vi "Unpack 32 i12s held in 24 i16s_lvfpga debug.vi"(8 "error in":errorcluster, 9 "destination i16 array":i16[](array[numeric])=[0, 16, 32, 48, 64, 80, 96, 112, 0, 0, 0, 0, 0, 0, 0, 0, 2064, 2320, 2576, 2832, 3088, 3344, 3600, 3856, 256, 256, 256, 256, 256, 256, 256, 256] format="%016b", 10 "packed i12s":i16[](array[numeric])=[0, 16, 32, 48, 64, 80, 96, 112, 2049, 2305, 2561, 2817, 3073, 3329, 3585, 3841, 24, 4121, 8218, 12315, 16412, 20509, 24606, 28703] format="%016b") -> (0 "error out":errorcluster, 1 "destination i16 array out":i16[](array[numeric])=[0, 16, 32, 48, 64, 80, 96, 112, 128, 144, 160, 176, 192, 208, 224, 240, -32768, -28656, -24544, -20432, -16320, -12208, -8096, -3984, 0, 256, 512, 768, 1024, 1280, 1536, 1792] format="%016b")   [LabVIEW 2012]
panel:
  out "destination i16 array (decimal)":i16[](array[numeric])
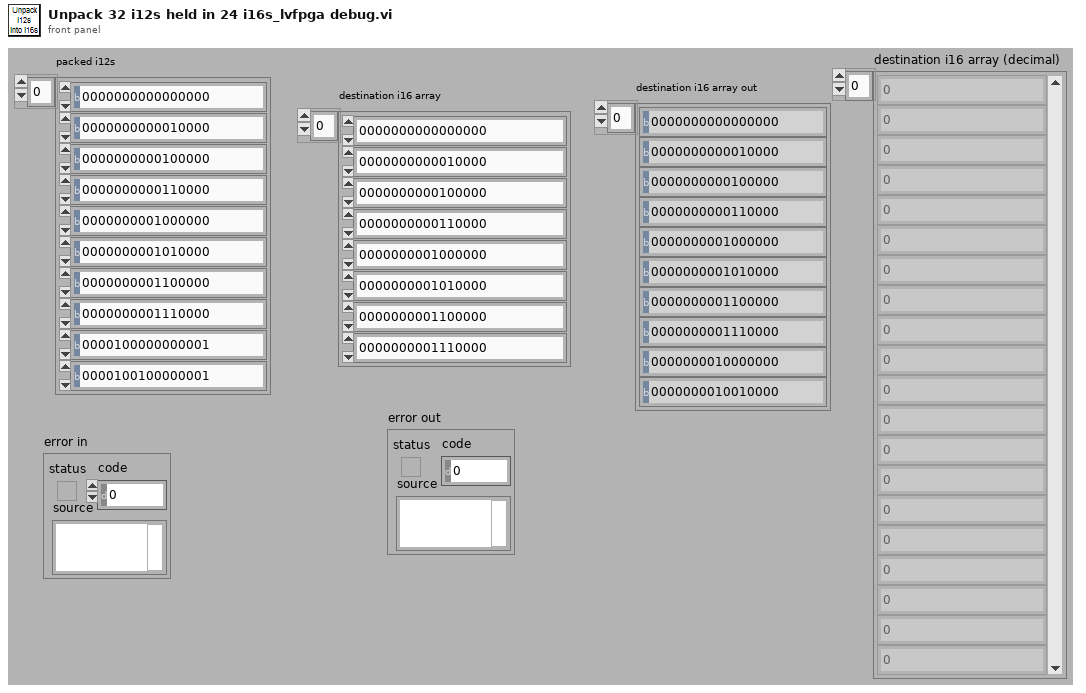
[diagram p1: front panel]
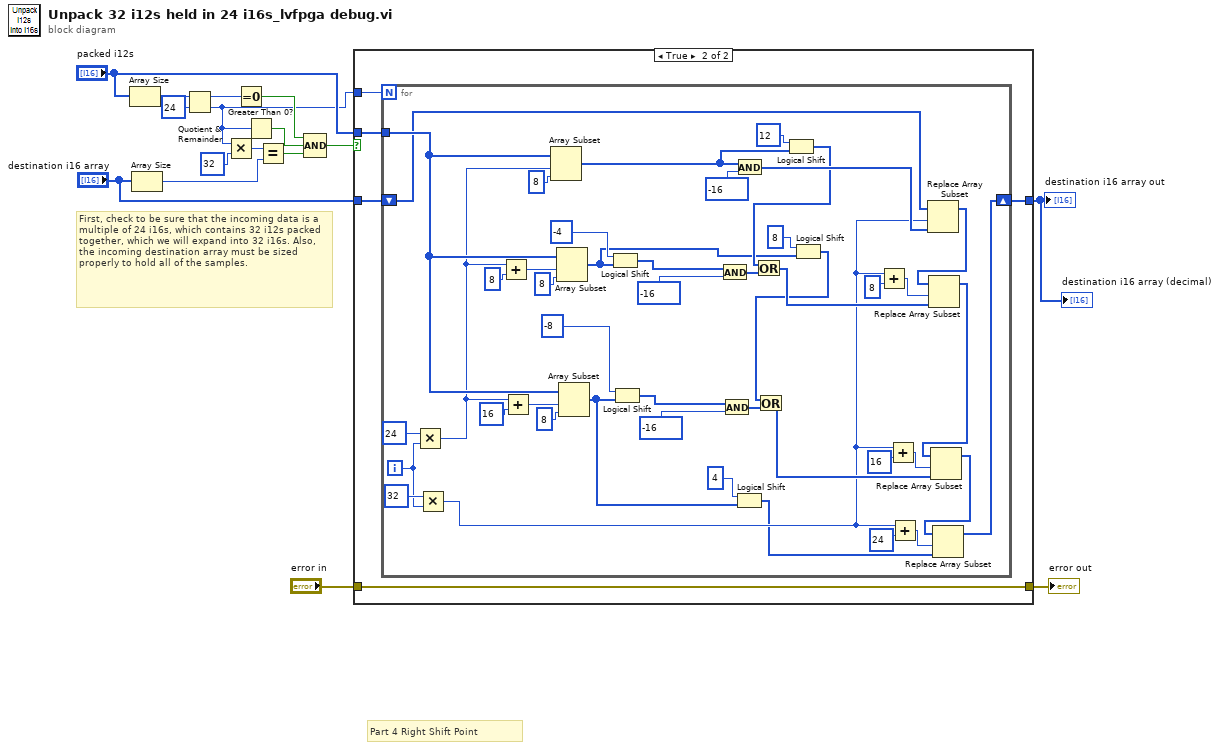
[diagram p0: block diagram]
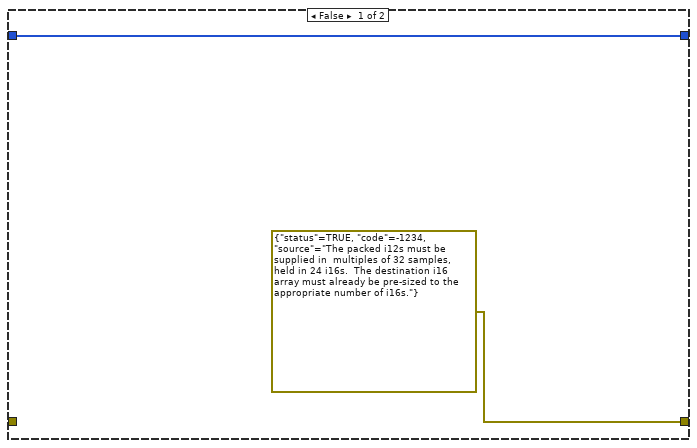
[diagram p2: hidden frame]
diagram:
  # "Part 4 Right Shift Point"
  # "First, check to be sure that the incoming data is a multiple of 24 i16s, which contains 32 i12s packed together, which we will expand into 32 i16s. Also, the incoming destination array must be sized properly to hold all of the samples."
  n1 = Array Size(array="packed i12s") -> (size(s)=w6:i32)
  n2 = Array Size(array="destination i16 array") -> (size(s)=w12:i32)
  n3 = Quotient & Remainder(x=w6, y=24) -> (x-y*floor(x/y)=w16:i32, floor(x/y)=w5:i32)
  n4 = Multiply(x=w5, y=32) -> (x*y=w13:i32)
  n5 = Equal To 0?(x=w16) -> (x = 0?=w11:bool)
  n6 = Greater Than 0?(x=w5) -> (x > 0?=w10:bool)
  n7 = Equal?(x=w13, y=w12) -> (x = y?=w9:bool)
  n8 = Compound Arithmetic op=AND(w11, w10, w9) -> (w7:bool)
  n9 = case shown="True" w7 {
    tunnel: "packed i12s" -> [_ w23]
    tunnel: w5 -> [_ w22]
    tunnel: "destination i16 array" -> [w18 w21]
    tunnel: [w18 w20] -> w3
    tunnel: [errorcluster {"status"=TRUE, "code"=-1234, "source"="The packed i12s must be supplied in  multiples of 32 samples, held in 24 i16s.  The destination i16 array must already be pre-sized to the appropriate number of i16s."} ("error IO") w19] -> w1
    tunnel: "error in" -> [_ w19]
    frame False {
    }
    frame True {
      n10 = for {
        N: w22 -> [_]
        tunnel: w23 -> [w43]
        shift-right: [w28] -> w20
        shift-left: w21 -> [w42]
        i -> [w58]
        n11 = Multiply(x=24, y=w58) -> (x*y=w39:i32)
        n12 = Multiply(x=32, y=w58) -> (x*y=w30:i32)
        n13 = Add(x=w39, y=8 ("x")) -> (x+y=w53:i32)
        n14 = Add(x=w39, y=16 ("x")) -> (x+y=w48:i32)
        n15 = Array Subset(array=w43, index=w39, length=8) -> (w61:i16[])
        n16 = Array Subset(array=w43, index=w53, length=8) -> (w24:i16[])
        n17 = Array Subset(array=w43, index=w48, length=8) -> (w26:i16[])
        n18 = Logical Shift(y=i16 -4 ("x"), x=w24) -> (x << y=w38:i16[])
        n19 = Logical Shift(y=i16 -8 ("x"), x=w26) -> (x << y=w36:i16[])
        n20 = And(x=w38, y=i16 -16 ("mask for lowest 4 bits")) -> (x .and. y?=w56:i16[])
        n21 = And(x=w36, y=i16 -16 ("mask for lowest 4 bits")) -> (x .and. y?=w25:i16[])
        n22 = Logical Shift(y=4 ("x"), x=w26) -> (x << y=w29:i16[])
        n23 = And(x=w61, y=i16 -16 ("mask for lowest 4 bits")) -> (x .and. y?=w57:i16[])
        n24 = Logical Shift(y=12 ("x"), x=w61) -> (x << y=w55:i16[])
        n25 = Or(x=w55, y=w56) -> (x .or. y?=w51:i16[])
        n26 = Logical Shift(y=8 ("x"), x=w24) -> (x << y=w34:i16[])
        n27 = Or(x=w34, y=w25) -> (x .or. y?=w50:i16[])
        n28 = Add(x=w30, y=8 ("x")) -> (x+y=w52:i32)
        n29 = Add(x=w30, y=16 ("x")) -> (x+y=w49:i32)
        n30 = Add(x=w30, y=24 ("x")) -> (x+y=w33:i32)
        n31 = Replace Array Subset(array=w42, new element=w57, index=w30) -> (w41:i16[])
        n32 = Replace Array Subset(array=w41, new element=w51, index=w52) -> (w40:i16[])
        n33 = Replace Array Subset(array=w40, new element=w50, index=w49) -> (w32:i16[])
        n34 = Replace Array Subset(array=w32, new element=w29, index=w33) -> (w28:i16[])
      }
    }
  }
  "error out" <- w1
  "destination i16 array out" <- w3
  "destination i16 array (decimal)" <- w3
